vi "__ABB start.vi"() -> ()   [LabVIEW 2017]
uses:
  ABB global.vi
panel:
  out "Exit":bool
  in  "stop":bool
  in  "Continue Test":bool
  in  "View Test":bool
  in  "Enter":bool
  in  "Password":string caption="Type in Password, \nthen press 'Enter'"
  in  "New Test":bool
  in  "Configure":bool
  in  "Quit":bool
  # "MOTOR TEST"
  # "Version 4.3"
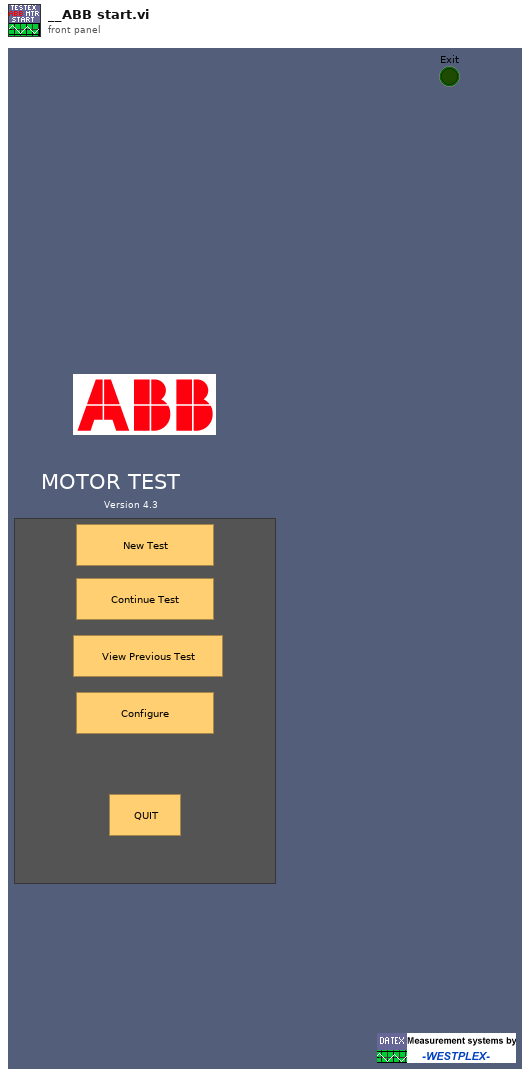
[diagram p1: front panel]
types:
  T1 = enum32{"existing file", "new file", "new or existing file", "existing dir", "new dir", "new or existing dir", "existing file (use LLBs)", "new file (use LLBs)", "new or existing file (use LLBs)", "new or existing file or directory (use LLBs)"}
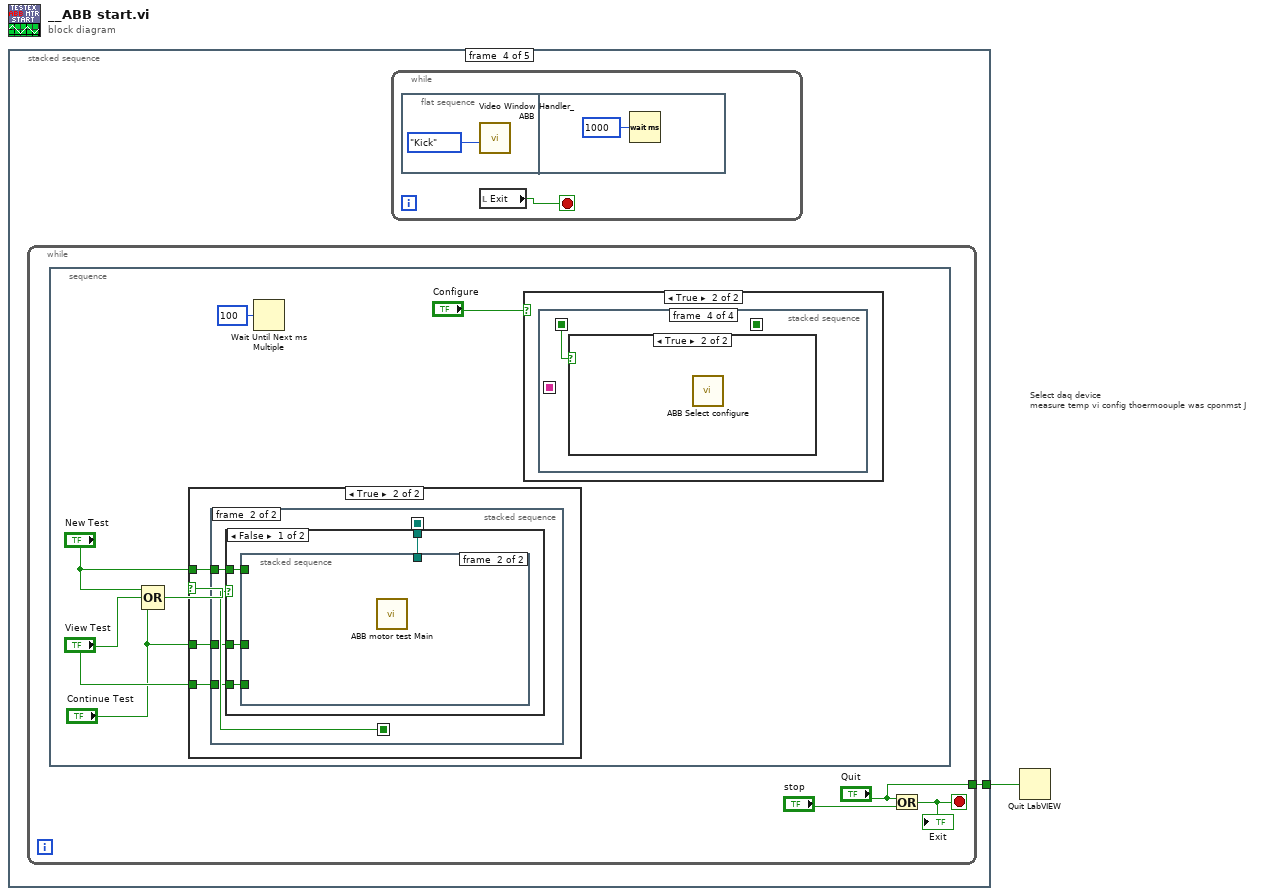
[diagram p0: block diagram]
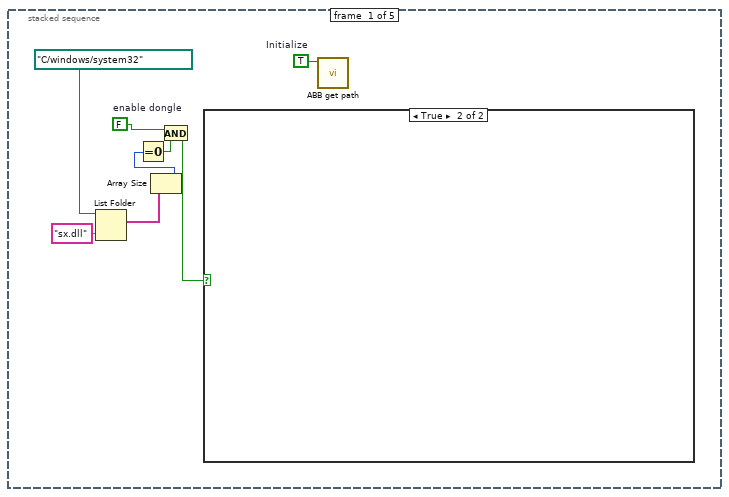
[diagram p2: hidden frame]
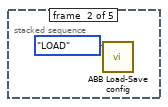
[diagram p4: hidden frame]
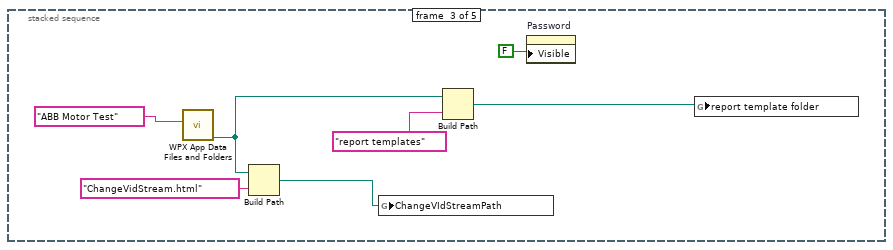
[diagram p5: hidden frame]
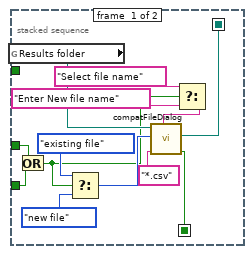
[diagram p7: hidden frame]
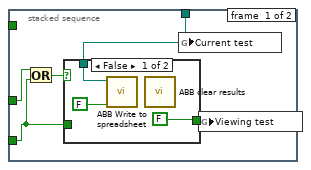
[diagram p8: hidden frame]
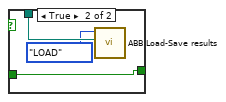
[diagram p9: hidden frame]
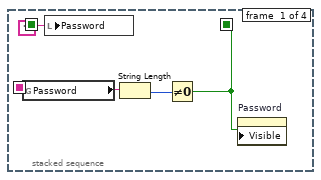
[diagram p12: hidden frame]
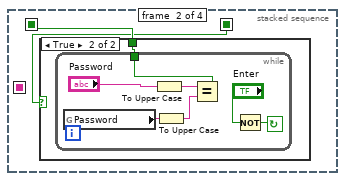
[diagram p13: hidden frame]
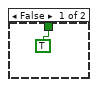
[diagram p14: hidden frame]
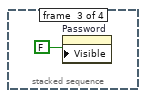
[diagram p15: hidden frame]
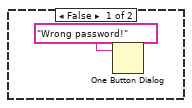
[diagram p16: hidden frame]
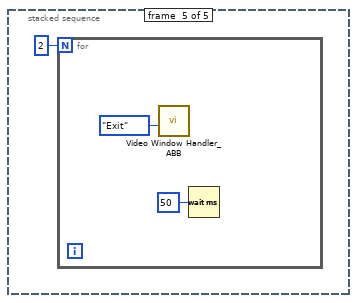
[diagram p17: hidden frame]
diagram:
  # "Select daq device\nmeasure temp vi config thoermoouple was cponmst J"
  n1 = stacked-sequence {
    tunnel: [_ _ _ w18 _] -> w1
    frame #0 {
      w2 = TRUE  # Initialize
      w5 = FALSE  # enable dongle
      n2 = List Folder(path=path "C:/windows/system32", pattern="sx.dll") -> (filenames=w8:string[])  [unwired: 2 in, 3 out]
      n3 = Array Size(array=w8) -> (size(s)=w7:i32)
      n4 = Equal To 0?(x=w7) -> (x = 0?=w6:bool)
      n5 = And(x=w5, y=w6) -> (x .and. y?=w3:bool)
      n6 = case shown="True" w3 {
        frame False {
        }
        frame True {
        }
      }
      n7 = call "ABB get path.vi"("Initialize"=w2) -> ()  [unwired: 10 in, 1 out]
    }
    frame #1 {
      n8 = call "ABB Load-Save config.vi"("Mode"=enum16{"LOAD", "SAVE"}."LOAD") -> ()  [unwired: 11 in]
    }
    frame #2 {
      n9 = call "WPX App Data Files and Folders.vi"("ApplicationName"="ABB Motor Test") -> ("DataFolder"=w13:path)  [unwired: 7 in, 3 out]
      n10 = Build Path(base path=w13, name or relative path="ChangeVidStream.html") -> (appended path=w11:path)
      n11 = global write "ABB global.vi" "ChangeVIdStreamPath"(w11) -> ()
      n12 = Build Path(base path=w13, name or relative path="report templates") -> (appended path=w16:path)
      n13 = property on="Password" class="Str"("Visible"=FALSE) -> ()  [unwired: 2 in, 2 out]
      n14 = global write "ABB global.vi" "report template folder"(w16) -> ()
    }
    frame #3 {
      n15 = while {
        tunnel: ["Quit"] -> w18
        stop <- w24 stop-if-true
        n16 = stacked-sequence {
          frame #0 {
            n17 = Compound Arithmetic op=OR("New Test", "View Test", "Continue Test") -> (w28:bool)
            n18 = case shown="True" w28 {
              tunnel: "View Test" -> [_ w33]
              tunnel: "Continue Test" -> [_ w32]
              tunnel: "New Test" -> [_ w31]
              frame False {
              }
              frame True {
                n19 = stacked-sequence {
                  seq-local: [w44 _] -> [_ w50]
                  seq-local: [w43 _] -> [_ w51]
                  tunnel: w33 -> [w37 w49]
                  tunnel: w32 -> [w35 w48]
                  tunnel: w31 -> [_ w47]
                  frame #0 {
                    n20 = global read "ABB global.vi" "Results folder"() -> (w45:path)
                    n21 = Or(x=w35, y=w37) -> (x .or. y?=w34:bool)
                    n22 = Select(t=T1."existing file", s=w34, f=T1."new file" ("select mode (2)")) -> (s? t:f=w41:T1)
                    n23 = Select(t="Select file name", s=w34, f="Enter New file name" ("prompt")) -> (s? t:f=w38:string)
                    n24 = call <vilib>:"compatFileDialog.vi"("prompt"=w38, "pattern"="*.csv", "select mode (2)"=w41, "start path"=w45) -> ("cancelled"=w43:bool, "path"=w44:path)  [unwired: 5 in, 1 out]
                  }
                  frame #1 {
                    n25 = case shown="False" w51 {
                      tunnel: w50 -> [w55 _]
                      tunnel: w49 -> [w54 _]
                      tunnel: w48 -> [w53 _]
                      tunnel: w47 -> [w52 _]
                      frame False {
                        n26 = stacked-sequence {
                          tunnel: w55 -> [w60 _]
                          tunnel: w54 -> [w56 _]
                          tunnel: w53 -> [w57 _]
                          tunnel: w52 -> [_ _]
                          frame #0 {
                            n27 = Or(x=w57, y=w56) -> (x .or. y?=w58:bool)
                            n28 = case shown="False" w58 {
                              tunnel: w60 -> [w63 w66]
                              tunnel: [FALSE w64] -> w59
                              tunnel: w56 -> [_ w64]
                              frame False {
                                n29 = call "ABB Write to spreadsheet.vi"("append to file? (new file:F)"=FALSE, "file path (dialog if empty)"=w63) -> ()  [unwired: 6 in, 1 out]
                                n30 = call "ABB clear results.vi"() -> ()  [unwired: 1 in]
                              }
                              frame True {
                                n31 = call "ABB Load-Save results.vi"("Path"=w66, "Mode"=enum16{"LOAD", "Save"}."LOAD") -> ()  [unwired: 10 in]
                              }
                            }
                            n32 = global write "ABB global.vi" "Current test"(w60) -> ()
                            n33 = global write "ABB global.vi" "Viewing test"(w59) -> ()
                          }
                          frame #1 {
                            n34 = call "ABB motor test Main.vi"() -> ()  [unwired: 1 in]
                          }
                        }
                      }
                      frame True {
                      }
                    }
                  }
                }
              }
            }
            n35 = Wait Until Next ms Multiple(millisecond multiple=u32 100) -> ()  [unwired: 1 out]
            n36 = case shown="True" "Configure" {
              frame False {
              }
              frame True {
                n37 = stacked-sequence {
                  seq-local: [_ w72 _ _] -> [_ _ _ w83]
                  seq-local: [w69 _ _ _] -> [_ _ _ _]
                  seq-local: [w67 _ _ _] -> [_ w71 _ _]
                  frame #0 {
                    n38 = global read "ABB global.vi" "Password"() -> (w69:string)
                    n39 = local write "Password"("") -> ()
                    n40 = String Length(string=w69) -> (length=w68:i32)
                    n41 = Not Equal To 0?(x=w68) -> (x != 0?=w67:bool)
                    n42 = property on="Password" class="Str"("Visible"=w67) -> ()  [unwired: 2 in, 2 out]
                  }
                  frame #1 {
                    n43 = case shown="True" w71 {
                      tunnel: [TRUE w74] -> w72
                      frame False {
                      }
                      frame True {
                        n44 = while {
                          tunnel: [w79] -> w74
                          stop <- w80 continue-if-true
                          n45 = global read "ABB global.vi" "Password"() -> (w81:string)
                          n46 = To Upper Case(1:"Password") -> (0:w77:string)
                          n47 = To Upper Case(1:w81) -> (0:w76:string)
                          n48 = Equal?(x=w77, y=w76) -> (x = y?=w79:bool)
                          n49 = Not(x="Enter") -> (.not. x?=w80:bool)
                        }
                      }
                    }
                  }
                  frame #2 {
                    n50 = property on="Password" class="Str"("Visible"=FALSE ("Write Attribute")) -> ()  [unwired: 2 in, 2 out]
                  }
                  frame #3 {
                    n51 = case shown="True" w83 {
                      frame False {
                        n52 = One Button Dialog(message="Wrong password!") -> ()  [unwired: 1 in, 1 out]
                      }
                      frame True {
                        n53 = call "ABB Select configure.vi"() -> ()  [unwired: 12 in]
                      }
                    }
                  }
                }
              }
            }
          }
        }
        n54 = Or(x="Quit", y="stop") -> (x .or. y?=w24:bool)
        "Exit" <- w24
      }
      n55 = while {
        stop <- w19 stop-if-true
        n56 = flat-sequence {
          frame #0 {
            n57 = call "Video Window Handler_ABB.vi"("Action"=enum16{"Show", "Hide", "Exit", "Kick"}."Kick") -> ()  [unwired: 11 in]
          }
          frame #1 {
            n58 = Wait (ms)(milliseconds to wait=u32 1000) -> ()  [unwired: 1 out]
          }
        }
        n59 = local read "Exit"() -> (w19:bool)
      }
    }
    frame #4 {
      n60 = for {
        N: 2 -> [_]
        n61 = call "Video Window Handler_ABB.vi"("Action"=enum16{"Show", "Hide", "Exit"}."Exit") -> ()  [unwired: 11 in]
        n62 = Wait (ms)(milliseconds to wait=u32 50) -> ()  [unwired: 1 out]
      }
    }
  }
  n63 = Quit LabVIEW(quit? (T)=w1) -> ()
